vi "Joysticks to Drive Motors.vi"(8 "Boost?":bool, 9 "Turn":dbl, 10 "Throttle":dbl) -> (2 "Drive Motor Values":cluster{"Left Motor":dbl, "Right Motor":dbl})   [LabVIEW 2018]
uses:
  Robot Global Data.vi
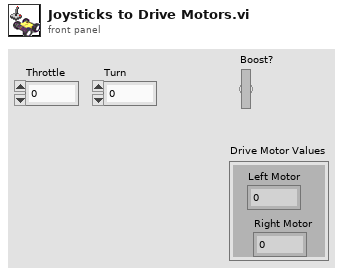
[diagram p1: front panel]
types:
  T1 = cluster{"Left Motor Value":dbl, "Right Motor Value":dbl}
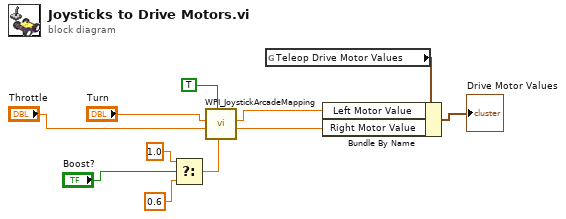
[diagram p0: block diagram]
diagram:
  n1 = Select(t=1.0 ("Max Output"), s="Boost?", f=0.6 ("Max Output")) -> (s? t:f=w11:dbl)
  n2 = call <vilib>:"WPI_JoystickArcadeMapping.vi"("Max Output"=w11, "Square Inputs"=TRUE, "Y axis value"="Throttle", "X axis value"="Turn") -> ("Right Motor Value"=w2:dbl, "Left Motor Value"=w3:dbl)  [unwired: 6 in]
  n3 = global read "Robot Global Data.vi" "Teleop Drive Motor Values"() -> (w4:T1)
  n4 = Bundle By Name(cluster=w4, "Left Motor Value"=w3, "Right Motor Value"=w2) -> (→"Drive Motor Values":T1)
